vi "Transmit Data To Aircraft.vi"(8 "Error In":errorcluster) -> ()   [LabVIEW 2014]
uses:
  Aircraft Data Router/Controls/Known Aircraft.ctl
  Controls/Coms Driver Interface.ctl
  Telemetry/Controls/Telemetry Connection Type.ctl
  <vilib>/httpClient/ClientHandle.ctl
  Web Services/DronePi Global Variables.vi
  <vilib>/httpClient/LabVIEWHTTPClient.lvlib
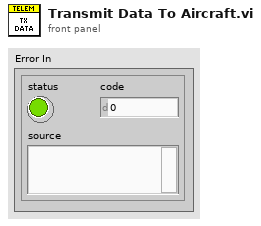
[diagram p1: front panel]
types:
  T1 = typedef "Known Aircraft.ctl" = cluster{"Aircraft ID":u8, "Aircraft Receive queue Ref":refnum<queue>, "Aircraft Transmit queue Ref":refnum<queue>, "Waypoint Queue Ref":refnum<queue>, "Connection Details":T2}
  T2 = typedef "Coms Driver Interface.ctl" = cluster{"Connection Type":T3, "UDP connection ID":refnum<k16>, "Serial COM port ID":refnum<visa-resource-name>, "IP Address of Aircraft":u32, "Remote Master Details":cluster{"Remote Master client handle":T4, "Base Path of Web Service":string}, "UDP TX Port of Aircraft":u16}
  T3 = typedef "Telemetry Connection Type.ctl" = enum16{"Serial", "UDP", "Remote Master"}
  T4 = typedef "LabVIEWHTTPClient.lvlib/ClientHandle.ctl" = refnum<k1>
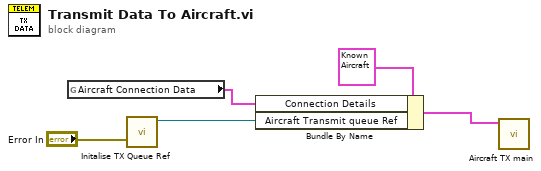
[diagram p0: block diagram]
diagram:
  n1 = global read "DronePi Global Variables.vi" "Aircraft Connection Data"() -> (w2:T2)
  n2 = call "Initalise TX Queue Ref.vi"("Error In"="Error In") -> ("TX Queue Out"=w3:refnum<queue>)  [unwired: 9 in, 1 out]
  n3 = Bundle By Name(cluster=T1 {"Aircraft ID"=0, "Aircraft Receive queue Ref"=refnum, "Aircraft Transmit queue Ref"=refnum, "Waypoint Queue Ref"=refnum, "Connection Details"={"Connection Type"=enum."Serial", "UDP connection ID"=refnum, "Serial COM port ID"="", "IP Address of Aircraft"=0, "Remote Master Details"={"Remote Master client handle"=refnum, "Base Path of Web Service"=""}, "UDP TX Port of Aircraft"=0}} ("Instance Details"), "Connection Details"=w2, "Aircraft Transmit queue Ref"=w3) -> (w1:T1)
  n4 = call "Aircraft TX main.vi"("Instance Details"=w1) -> ()  [unwired: 11 in]
